vi "Auto-adjust line length.vi"(6 "Equal size":bool, 7 "Current ROI Tool":i32, 8 "error in (no error)":errorcluster, 11 "New Coordinates":i32[](array[numeric])) -> (0 "error out":errorcluster, 1 "Do not generate ROI":bool, 3 "Output coordinates":i32[](array[numeric]))   [LabVIEW 2017]
panel:
  # "X1\nY1\nX2\nY2"
  # "X1\nY1\nX2\nY2"
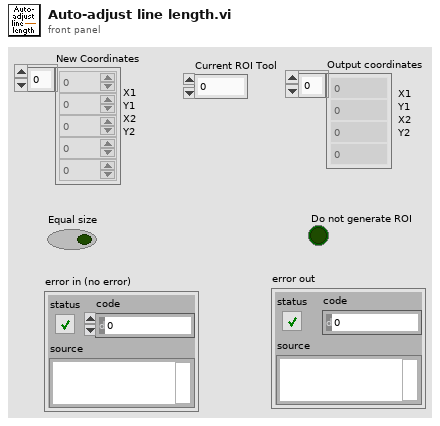
[diagram p1: front panel]
types:
  T1 = typedef "Line draw mode.ctl" = enum16{"Free draw", "Orthogonal"}
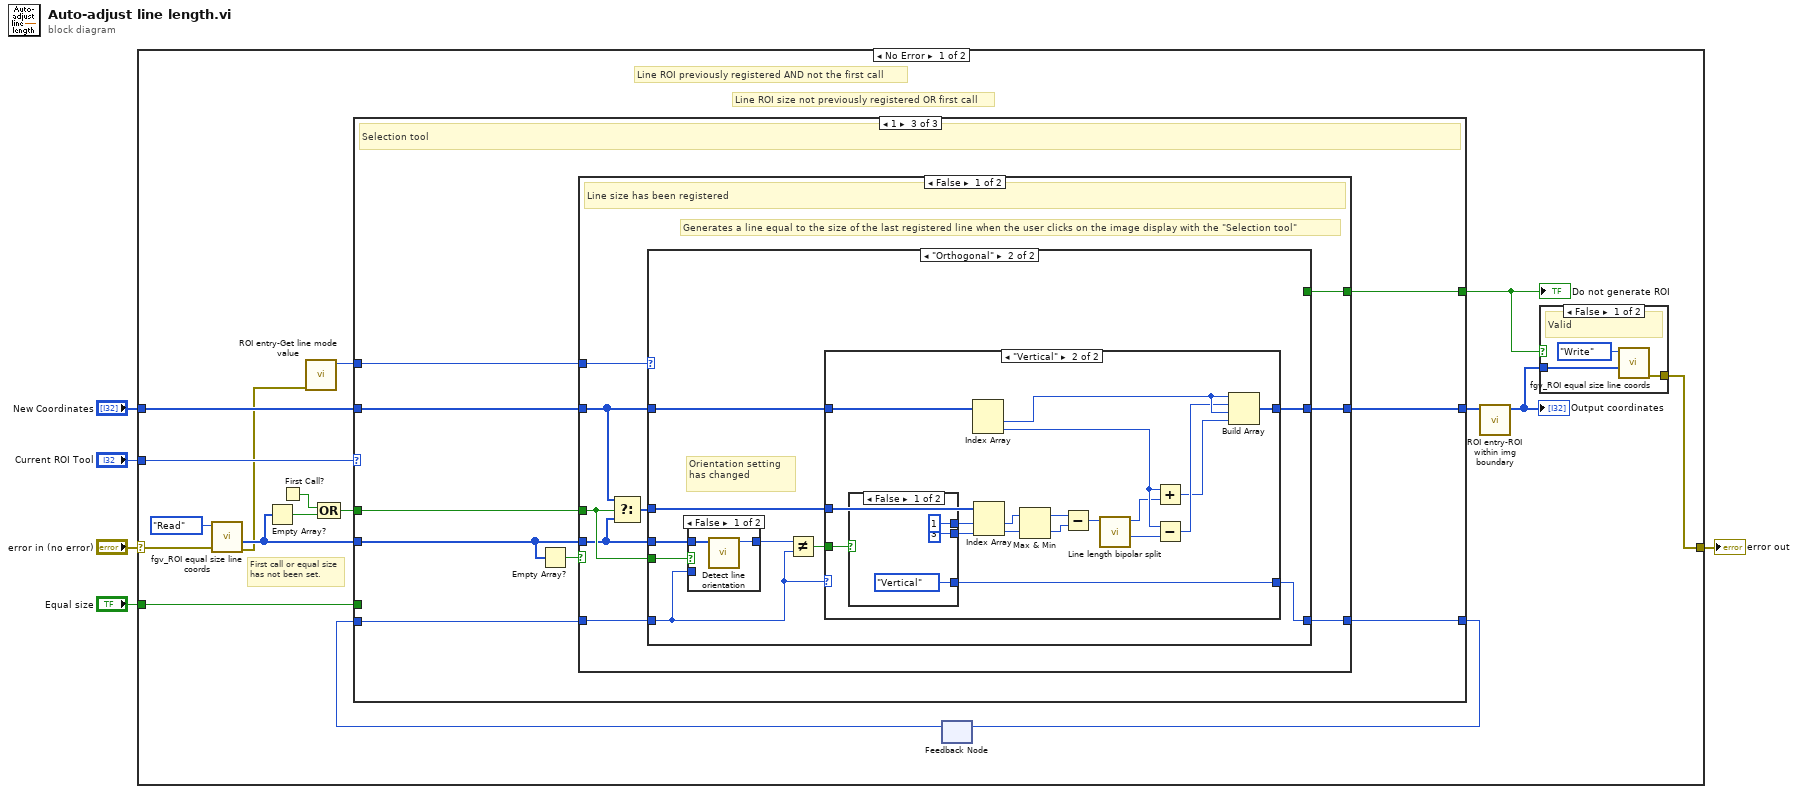
[diagram p0: block diagram]
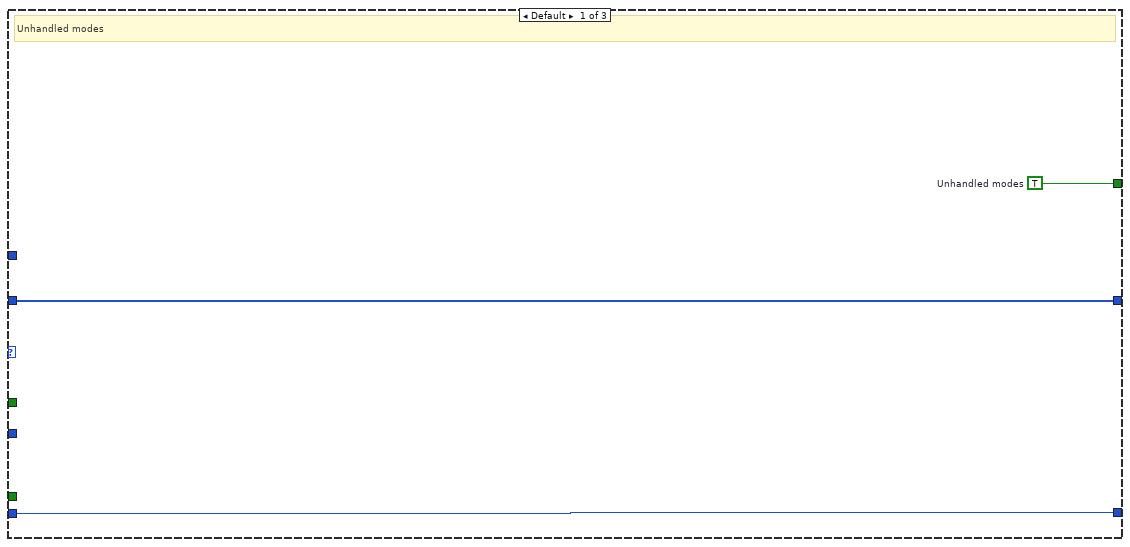
[diagram p3: hidden frame]
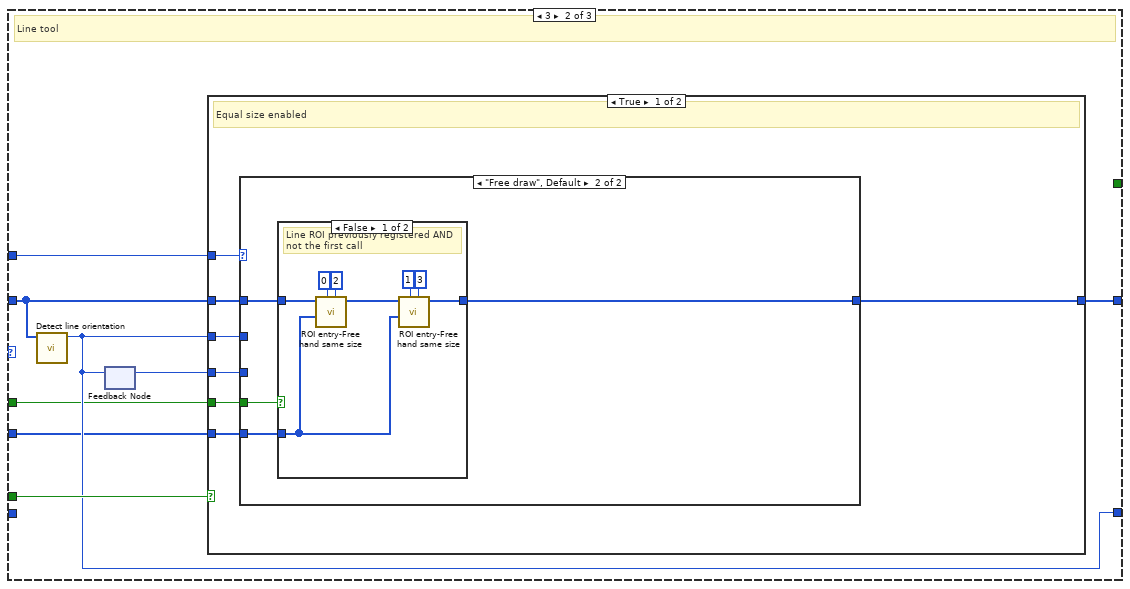
[diagram p4: hidden frame]
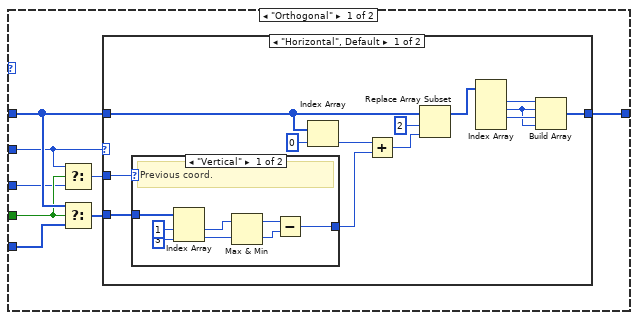
[diagram p5: hidden frame]
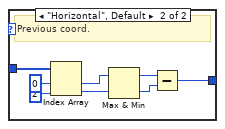
[diagram p6: hidden frame]
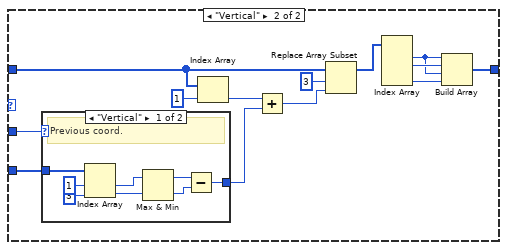
[diagram p7: hidden frame]
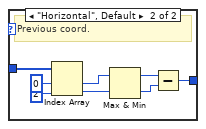
[diagram p8: hidden frame]
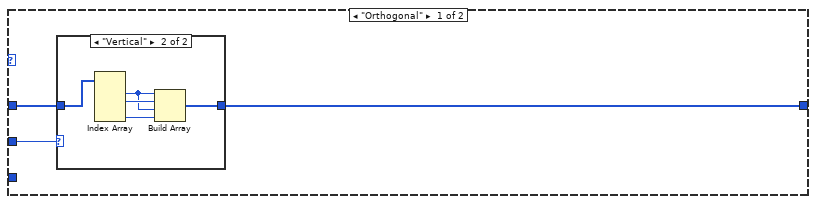
[diagram p11: hidden frame]
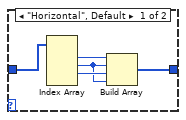
[diagram p12: hidden frame]
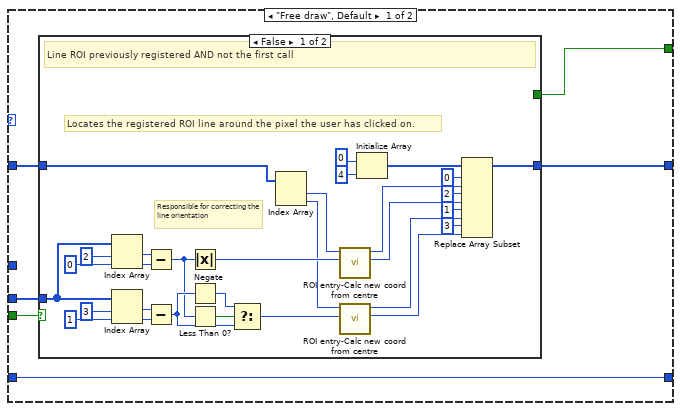
[diagram p13: hidden frame]
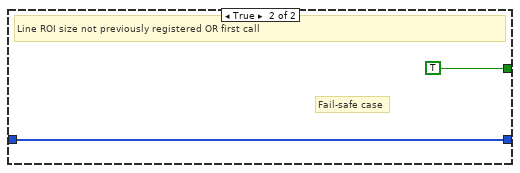
[diagram p14: hidden frame]
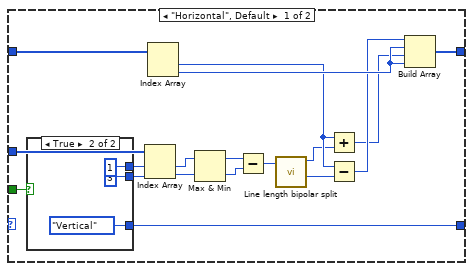
[diagram p16: hidden frame]
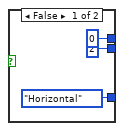
[diagram p17: hidden frame]
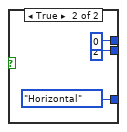
[diagram p18: hidden frame]
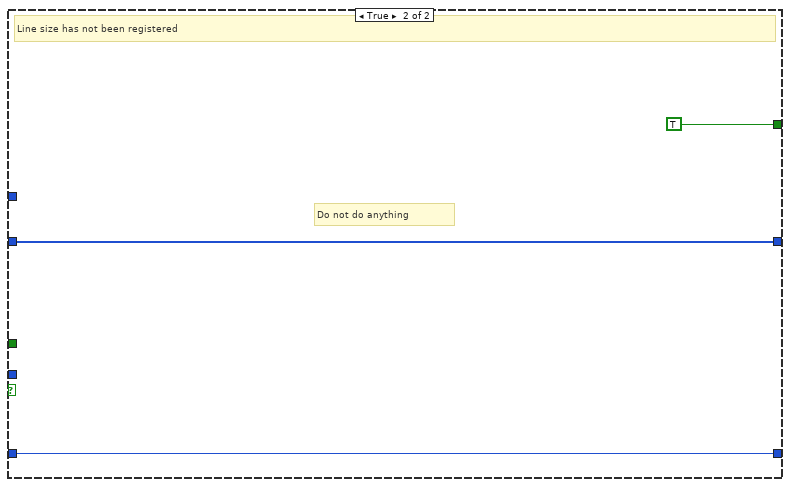
[diagram p19: hidden frame]
diagram:
  n1 = case shown="No Error" "error in (no error)" {
    selector: "error in (no error)" -> [w8 w263]
    tunnel: "New Coordinates" -> [w22 _]
    tunnel: "Current ROI Tool" -> [w19 _]
    tunnel: "Equal size" -> [w18 _]
    tunnel: [w6 w263] -> w1
    frame No Error {
      # "Line ROI size not previously registered OR first call"
      # "Line ROI previously registered AND not the first call"
      # "First call or equal size has not been set."
      n2 = call "fgv_ROI equal size line coords.vi"("error in (no error)"=w8, "Function"=enum16{"Intialize", "Write", "Read", "Clear"}."Read") -> ("error out"=w7:errorcluster, "Registered Line Coordinates"=w12:i32[])  [unwired: 8 in]
      n3 = Empty Array?(array=w12) -> (empty?=w13:bool)
      n4 = First Call?() -> (First Call?: T/F=w16:bool)
      n5 = call "ROI entry-Get line mode value.vi"("error in (no error)"=w7) -> ("Drawing Mode setting"=w15:T1)  [unwired: 9 in, 1 out]
      n6 = Compound Arithmetic op=OR(w16, w13) -> (w17:bool)
      n7 = feedback #1() -> (w20:enum16{"Horizontal", "Vertical"})  [unwired: 1 in]
      n8 = case shown="1" w19 {
        tunnel: w18 -> [_ w36 _]
        tunnel: w17 -> [_ w30 w152]
        tunnel: w15 -> [_ w34 w151]
        tunnel: w22 -> [w28 w33 w150]
        tunnel: [w28 w29 w149] -> w10
        tunnel: w12 -> [_ w31 w147]
        tunnel: [w27 w32 w144] -> w21
        tunnel: w20 -> [w27 _ w145]
        tunnel: [w26 _ w148] -> w9
        frame Default {
          w26 = TRUE  # Unhandled modes
          # "Unhandled modes"
        }
        frame 3 {
          # "Line tool"
          n9 = call "Detect line orientation.vi"("Coordinates"=w33) -> ("Vertical or Horisontal?"=w32:enum16{"Horizontal", "Vertical"})  [unwired: 10 in]
          n10 = feedback #2() -> (w35:enum16{"Horizontal", "Vertical"})  [unwired: 1 in]
          n11 = feedback-in #2(w32) -> ()
          n12 = case shown="True" w36 {
            tunnel: w33 -> [w43 w129]
            tunnel: w32 -> [w40 w126]
            tunnel: w35 -> [w39 w125]
            tunnel: w34 -> [w37 w123]
            tunnel: [w38 w124] -> w29
            tunnel: w31 -> [w42 w128]
            tunnel: w30 -> [w41 w127]
            frame True {
              # "Equal size enabled"
              n13 = case shown="\"Free draw\", Default" w37 {
                tunnel: w43 -> [w51 w113]
                tunnel: w42 -> [w50 w110]
                tunnel: w41 -> [w48 w111]
                tunnel: w40 -> [w47 _]
                tunnel: w39 -> [w46 _]
                tunnel: [w44 w112] -> w38
                frame "Orthogonal" {
                  n14 = Select(t=w47, s=w48, f=w46) -> (s? t:f=w45:enum16{"Horizontal", "Vertical"})
                  n15 = Select(t=w51, s=w48, f=w50) -> (s? t:f=w49:i32[])
                  n16 = case shown="\"Horizontal\", Default" w47 {
                    tunnel: w51 -> [w62 w90]
                    tunnel: w49 -> [w59 w93]
                    tunnel: w45 -> [w58 w86]
                    tunnel: [w52 w81] -> w44
                    frame "Horizontal", Default {
                      n17 = case shown="\"Vertical\"" w58 {
                        tunnel: w59 -> [w66 w74]
                        tunnel: [w65 w73] -> w57
                        frame "Vertical" {
                          # "Previous coord."
                          n18 = Index Array(array=w66, index #1=1 ("index"), index #2=3 ("index")) -> (element #1=w70:i32, element #2=w69:i32)
                          n19 = Max & Min(x=w70, y=w69) -> (max(x,y)=w68:i32, min(x,y)=w67:i32)
                          n20 = Subtract(x=w68, y=w67) -> (x-y=w65:i32)
                        }
                        frame "Horizontal", Default {
                          # "Previous coord."
                          n21 = Index Array(array=w74, index #1=0 ("index"), index #2=2 ("index")) -> (element #1=w78:i32, element #2=w77:i32)
                          n22 = Max & Min(x=w78, y=w77) -> (max(x,y)=w76:i32, min(x,y)=w75:i32)
                          n23 = Subtract(x=w76, y=w75) -> (x-y=w73:i32)
                        }
                      }
                      n24 = Index Array(array=w62, index=0) -> (element=w63:i32)
                      n25 = Add(x=w63, y=w57) -> (x+y=w60:i32)
                      n26 = Replace Array Subset(array=w62, new element=w60, index=2) -> (w53:i32[])
                      n27 = Index Array(array=w53) -> (element #1=w55:i32, element #2=w54:i32, element #3=w56:i32)  [unwired: 4 in, 1 out]
                      n28 = Build Array(w55, w54, w56, w54) -> (w52:i32[])
                    }
                    frame "Vertical" {
                      n29 = case shown="\"Vertical\"" w86 {
                        tunnel: w93 -> [w95 w103]
                        tunnel: [w94 w102] -> w87
                        frame "Vertical" {
                          # "Previous coord."
                          n30 = Index Array(array=w95, index #1=1 ("index"), index #2=3 ("index")) -> (element #1=w99:i32, element #2=w98:i32)
                          n31 = Max & Min(x=w99, y=w98) -> (max(x,y)=w97:i32, min(x,y)=w96:i32)
                          n32 = Subtract(x=w97, y=w96) -> (x-y=w94:i32)
                        }
                        frame "Horizontal", Default {
                          # "Previous coord."
                          n33 = Index Array(array=w103, index #1=0 ("index"), index #2=2 ("index")) -> (element #1=w107:i32, element #2=w106:i32)
                          n34 = Max & Min(x=w107, y=w106) -> (max(x,y)=w105:i32, min(x,y)=w104:i32)
                          n35 = Subtract(x=w105, y=w104) -> (x-y=w102:i32)
                        }
                      }
                      n36 = Index Array(array=w90, index=1) -> (element=w91:i32)
                      n37 = Add(x=w91, y=w87) -> (x+y=w88:i32)
                      n38 = Replace Array Subset(array=w90, new element=w88, index=3) -> (w82:i32[])
                      n39 = Index Array(array=w82) -> (element #1=w83:i32, element #2=w84:i32, element #4=w85:i32)  [unwired: 4 in, 1 out]
                      n40 = Build Array(w83, w84, w83, w85) -> (w81:i32[])
                    }
                  }
                }
                frame "Free draw", Default {
                  n41 = case shown="False" w111 {
                    tunnel: w113 -> [w119 w122]
                    tunnel: [w117 w122] -> w112
                    tunnel: w110 -> [w114 _]
                    frame False {
                      # "Line ROI previously registered AND not the first call"
                      n42 = call "ROI entry-Free hand same size.vi"("Index of ROI end"=2 ("index"), "Index of ROI start"=0 ("index"), "Registered Line Coordinates"=w114, "Coordinates in"=w119) -> ("Coordinates out"=w118:i32[])  [unwired: 7 in]
                      n43 = call "ROI entry-Free hand same size.vi"("Index of ROI end"=3 ("index"), "Index of ROI start"=1 ("index"), "Registered Line Coordinates"=w114, "Coordinates in"=w118) -> ("Coordinates out"=w117:i32[])  [unwired: 7 in]
                    }
                    frame True {
                      # "Line ROI size not previously registered OR first call"
                    }
                  }
                }
              }
            }
            frame False {
              # "Equal size disabled"
              n44 = case shown="\"Free draw\", Default" w123 {
                tunnel: w129 -> [w130 w143]
                tunnel: w128 -> [_ _]
                tunnel: w127 -> [_ _]
                tunnel: w126 -> [w132 _]
                tunnel: w125 -> [_ _]
                tunnel: [w131 w143] -> w124
                frame "Orthogonal" {
                  n45 = case shown="\"Vertical\"" w132 {
                    tunnel: w130 -> [w133 w138]
                    tunnel: [w134 w139] -> w131
                    frame "Horizontal", Default {
                      n46 = Index Array(array=w133) -> (element #1=w136:i32, element #2=w135:i32, element #3=w137:i32)  [unwired: 4 in, 1 out]
                      n47 = Build Array(w136, w135, w137, w135) -> (w134:i32[])
                    }
                    frame "Vertical" {
                      n48 = Index Array(array=w138) -> (element #1=w140:i32, element #2=w141:i32, element #4=w142:i32)  [unwired: 4 in, 1 out]
                      n49 = Build Array(w140, w141, w140, w142) -> (w139:i32[])
                    }
                  }
                }
                frame "Free draw", Default {
                }
              }
            }
          }
        }
        frame 1 {
          # "Selection tool"
          n50 = Empty Array?(array=w147) -> (empty?=w146:bool)
          n51 = case shown="False" w146 {
            tunnel: w152 -> [w156 _]
            tunnel: w151 -> [w160 _]
            tunnel: w150 -> [w159 w261]
            tunnel: [w157 w261] -> w149
            tunnel: w147 -> [w155 _]
            tunnel: w145 -> [w158 w260]
            tunnel: [w154 TRUE] -> w148
            tunnel: [w153 w260] -> w144
            frame False {
              # "Generates a line equal to the size of the last registered line when the user clicks on the image display with the \"Selection tool\""
              # "Line size has been registered"
              n52 = Select(t=w159, s=w156, f=w155) -> (s? t:f=w161:i32[])
              n53 = case shown="\"Orthogonal\"" w160 {
                tunnel: w159 -> [w167 w208]
                tunnel: w161 -> [_ w207]
                tunnel: [w165 w206] -> w157
                tunnel: w158 -> [w162 w202]
                tunnel: w156 -> [w166 w205]
                tunnel: w155 -> [w164 w204]
                tunnel: [w163 _] -> w154
                tunnel: [w162 w200] -> w153
                frame "Free draw", Default {
                  n54 = case shown="False" w166 {
                    tunnel: w167 -> [w187 w199]
                    tunnel: [w189 w199] -> w165
                    tunnel: w164 -> [w188 _]
                    tunnel: [_ TRUE] -> w163
                    frame False {
                      # "Responsible for correcting the line orientation"
                      # "Locates the registered ROI line around the pixel the user has clicked on."
                      # "Line ROI previously registered AND not the first call"
                      n55 = Index Array(array=w188, index #1=2 ("index"), index #2=0 ("index")) -> (element #1=w195:i32, element #2=w194:i32)
                      n56 = Index Array(array=w188, index #1=3 ("index"), index #2=1 ("index")) -> (element #1=w192:i32, element #2=w193:i32)
                      n57 = Subtract(x=w195, y=w194) -> (x-y=w173:i32)
                      n58 = Subtract(x=w192, y=w193) -> (x-y=w174:i32)
                      n59 = Absolute Value(x=w173) -> (abs(x)=w172:i32)
                      n60 = Negate(x=w174) -> (-x=w176:i32)
                      n61 = Less Than 0?(x=w173) -> (x < 0?=w175:bool)
                      n62 = Select(t=w176, s=w175, f=w174) -> (s? t:f=w170:i32)
                      n63 = Index Array(array=w187) -> (element #1=w186:i32, element #2=w171:i32)  [unwired: 2 in]
                      n64 = call "ROI entry-Calc new coord from centre.vi"("Previous length"=w172, "Central point coordinate"=w186) -> ("New max"=w183:i32, "New min"=w185:i32)  [unwired: 8 in]
                      n65 = call "ROI entry-Calc new coord from centre.vi"("Previous length"=w170, "Central point coordinate"=w171) -> ("New max"=w168:i32, "New min"=w169:i32)  [unwired: 8 in]
                      n66 = Initialize Array(0 ("dimension size"), 4 ("dimension size")) -> (w177:i32[])
                      n67 = Replace Array Subset(array=w177, new element #1=w185, index #1=0 ("index"), new element #2=w183, index #2=2 ("index"), new element #3=w169, index #3=1 ("index"), new element #4=w168, index #4=3 ("index")) -> (w189:i32[])
                    }
                    frame True {
                      # "Fail-safe case"
                      # "Line ROI size not previously registered OR first call"
                    }
                  }
                }
                frame "Orthogonal" {
                  # "Orientation setting has changed"
                  n68 = case shown="False" w205 {
                    tunnel: w204 -> [w210 _]
                    tunnel: [w209 w211] -> w203
                    tunnel: w202 -> [_ w211]
                    frame False {
                      n69 = call "Detect line orientation.vi"("Coordinates"=w210) -> ("Vertical or Horisontal?"=w209:enum16{"Horizontal", "Vertical"})  [unwired: 10 in]
                    }
                    frame True {
                    }
                  }
                  n70 = Not Equal?(x=w203, y=w202) -> (x != y?=w201:bool)
                  n71 = case shown="\"Vertical\"" w202 {
                    tunnel: w208 -> [w229 w252]
                    tunnel: w207 -> [w228 w253]
                    tunnel: [w214 w238] -> w206
                    tunnel: w201 -> [w213 w237]
                    tunnel: [w212 w236] -> w200
                    frame "Horizontal", Default {
                      n72 = case shown="True" w213 {
                        tunnel: [0 ("index") 1 ("index")] -> w227
                        tunnel: [2 ("index") 3 ("index")] -> w226
                        tunnel: [enum16{"Horizontal", "Vertical"}."Horizontal" ("Vertical or Horisontal?") enum16{"Horizontal", "Vertical"}."Vertical" ("Vertical or Horisontal?")] -> w212
                        frame False {
                        }
                        frame True {
                        }
                      }
                      n73 = Index Array(array=w228, index #1=w227, index #2=w226) -> (element #1=w225:i32, element #2=w224:i32)
                      n74 = Index Array(array=w229) -> (element #1=w218:i32, element #2=w221:i32)  [unwired: 2 in]
                      n75 = Max & Min(x=w225, y=w224) -> (max(x,y)=w223:i32, min(x,y)=w222:i32)
                      n76 = Subtract(x=w223, y=w222) -> (x-y=w217:i32)
                      n77 = call "Line length bipolar split.vi"("Line length"=w217) -> ("Positive length"=w215:i32, "Negative length"=w216:i32)  [unwired: 9 in]
                      n78 = Add(x=w218, y=w216) -> (x+y=w219:i32)
                      n79 = Subtract(x=w218, y=w215) -> (x-y=w220:i32)
                      n80 = Build Array(w220, w221, w219, w221) -> (w214:i32[])
                    }
                    frame "Vertical" {
                      n81 = case shown="False" w237 {
                        tunnel: [1 ("index") 0 ("index")] -> w251
                        tunnel: [3 ("index") 2 ("index")] -> w250
                        tunnel: [enum16{"Horizontal", "Vertical"}."Vertical" ("Vertical or Horisontal?") enum16{"Horizontal", "Vertical"}."Horizontal" ("Vertical or Horisontal?")] -> w236
                        frame False {
                        }
                        frame True {
                        }
                      }
                      n82 = Index Array(array=w252) -> (element #1=w245:i32, element #2=w244:i32)  [unwired: 2 in]
                      n83 = Index Array(array=w253, index #1=w251, index #2=w250) -> (element #1=w249:i32, element #2=w248:i32)
                      n84 = Max & Min(x=w249, y=w248) -> (max(x,y)=w247:i32, min(x,y)=w246:i32)
                      n85 = Subtract(x=w247, y=w246) -> (x-y=w241:i32)
                      n86 = call "Line length bipolar split.vi"("Line length"=w241) -> ("Positive length"=w239:i32, "Negative length"=w240:i32)  [unwired: 9 in]
                      n87 = Add(x=w244, y=w240) -> (x+y=w242:i32)
                      n88 = Subtract(x=w244, y=w239) -> (x-y=w243:i32)
                      n89 = Build Array(w245, w243, w245, w242) -> (w238:i32[])
                    }
                  }
                }
              }
            }
            frame True {
              # "Do not do anything"
              # "Line size has not been registered"
            }
          }
        }
      }
      "Do not generate ROI" <- w9
      n90 = feedback-in #1(w21) -> ()
      n91 = call "ROI entry-ROI within img boundary.vi"("Coordinates in"=w10) -> ("Coordinates out"=w11:i32[])  [unwired: 10 in]
      "Output coordinates" <- w11
      n92 = case shown="False" w9 {
        tunnel: w11 -> [w24 _]
        tunnel: [w23 _] -> w6
        frame False {
          # "Valid"
          n93 = call "fgv_ROI equal size line coords.vi"("New Line Coordinates"=w24, "Function"=enum16{"Intialize", "Write", "Read", "Clear"}."Write") -> ("error out"=w23:errorcluster)  [unwired: 8 in, 1 out]
        }
        frame True {
          # "Invalid"
        }
      }
    }
    frame Error {
    }
  }
  "error out" <- w1
